vi "draw_temporal_calibration.vi"(4 "TC One XY values (Projector Pixels)":i32[][](array[numeric]), 5 "Other Bits To Be Encoded":bool[](array[boolean]), 6 "TC Zero XY values (Projector Pixels)":i32[][](array[numeric]), 7 "error in (no error)":errorcluster, 8 "Buffer  Bits To Be Encoded":bool[](array[boolean]), 9 "TC Dot Radius (Projector Pixels)":i32, 10 "Image in":T1) -> (0 "error out":errorcluster, 3 "Image Out":T1)   [LabVIEW 2019]
uses:
  <vilib>/vision/Image Controls.llb/IMAQ Image.ctl
  <vilib>/vision/NI_Vision_Development_Module.lvlib
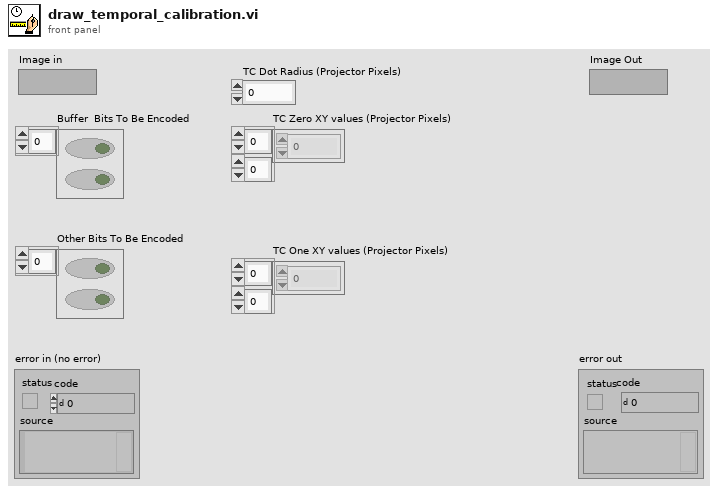
[diagram p1: front panel]
types:
  T1 = typedef "IMAQ Image.ctl" = refnum<image>
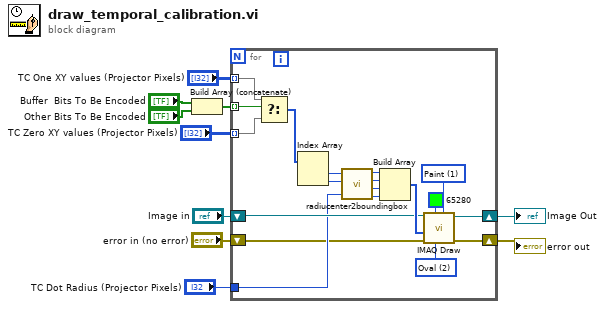
[diagram p0: block diagram]
diagram:
  n1 = Build Array (concatenate)("Buffer  Bits To Be Encoded", "Other Bits To Be Encoded") -> (w6:bool[])
  n2 = for {
    shift-right: [w21] -> w10
    shift-left: "Image in" -> [w22]
    shift-right: [w20] -> w9
    shift-left: "error in (no error)" -> [w17]
    tunnel: w6 -> [w19] mode=indexing
    tunnel: "TC Dot Radius (Projector Pixels)" -> [w18]
    tunnel: "TC One XY values (Projector Pixels)" -> [w16] mode=indexing
    tunnel: "TC Zero XY values (Projector Pixels)" -> [w15] mode=indexing
    w29 = u16 1 items=["Frame", "Paint", "Invert Frame", "Invert Paint"] ("Draw Mode")
    w28 = u16 2 items=["Line", "Rectangle", "Oval"] ("Shape to draw")
    n3 = Select(t=w16, s=w19, f=w15) -> (s? t:f=w14:i32[])
    n4 = Index Array(array=w14) -> (element #1=w13:i32, element #2=w12:i32)  [unwired: 2 in]
    n5 = call "radiucenter2boundingbox.vi"("Radius"=w18, "ycenter"=w12, "xcenter"=w13) -> ("Bottom"=w23:i32, "Right"=w24:i32, "Top"=w25:i32, "Left"=w26:i32)  [unwired: 2 in]
    n6 = Build Array(w26, w25, w24, w23) -> (w27:i32[])
    n7 = call "IMAQ Draw"("Draw Mode"=w29, "Shape to draw"=w28, "Pixel Color"=u32 65280 ("Color Pixel Value"), "error in (no error)"=w17, "Coordinates"=w27, "Image Src"=w22) -> ("error out"=w20:errorcluster, "Image Dst Out"=w21:T1)  [unwired: 4 in]
  }
  "Image Out" <- w10
  "error out" <- w9
